vi "Read Ctl Refnum.vi"(4 "Error In":errorcluster, 7 "Font Settting in":refnum<class "Display Properties.lvclass">) -> (0 "Error Out":errorcluster, 2 "Ctl Refnum":refnum<vi>, 3 "Font Settting out":refnum<class "Display Properties.lvclass">)   [LabVIEW 2015, in "Display Properties Manager.lvlib" / "Display Properties.lvclass"]
uses:
  Display Properties.lvclass
  Display Properties.lvclass/Display Properties.ctl
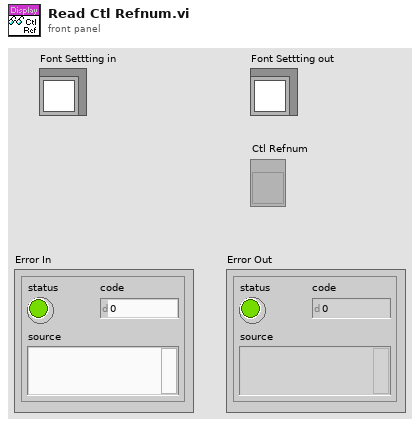
[diagram p1: front panel]
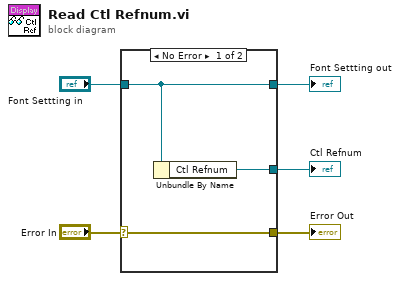
[diagram p0: block diagram]
diagram:
  n1 = case shown="No Error" "Error In" {
    selector: "Error In" -> [w8 w9]
    tunnel: [w8 w9] -> w4
    tunnel: [w7 w10] -> w2
    tunnel: "Font Settting in" -> [w7 w10]
    tunnel: [w6 _] -> w1
    frame No Error {
      n2 = Unbundle By Name(w7) -> ("Ctl Refnum"=w6:refnum<vi>)
    }
    frame Error {
    }
  }
  "Error Out" <- w4
  "Font Settting out" <- w2
  "Ctl Refnum" <- w1
